vi "private_data (library_variable).vi"() -> ()   [LabVIEW 2020, in "text_file.lvlib"]
uses:
  text_file.lvlib
panel:
  in  "text file refnum":refnum<file>
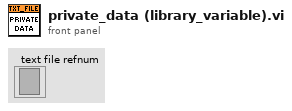
[diagram p1: front panel]
diagram:
